vi "detector_acquire_generic_data.vi"(8 "error in (no error)":errorcluster, 11 "picoquant_generic in":refnum<class "picoquant_generic.lvclass">) -> (0 "error out":errorcluster, 2 "image_data":T1, 3 "picoquant_generic out":refnum<class "picoquant_generic.lvclass">)   [LabVIEW 2015, in "picoquant_generic.lvclass"]
uses:
  picoquant_generic.lvclass
  Experiment/experiment_panel/2d_scan/detector_data_tdef.ctl
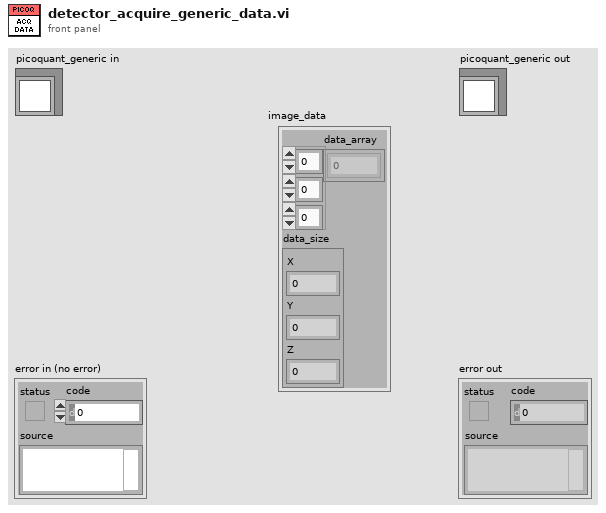
[diagram p1: front panel]
types:
  T1 = typedef "detector_data_tdef.ctl" = cluster{"data_array":dbl[][][], "data_size":cluster{"X":i32, "Y":i32, "Z":i32}}
  T2 = typedef "hydraharp_count_rates.ctl" = cluster{"channel_rates":i32[], "sync_rate":i32}
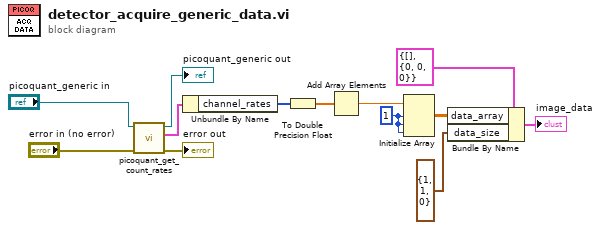
[diagram p0: block diagram]
diagram:
  w1 = 1 ("dimension size")
  n1 = call-dynamic "picoquant_get_count_rates.vi"("error in (no error)"="error in (no error)", "picoquant_generic in"="picoquant_generic in") -> ("error out"=→"error out":errorcluster, "count_rates"=w10:T2, "picoquant_generic out"=→"picoquant_generic out":refnum<class "picoquant_generic.lvclass">)  [unwired: 7 in]
  n2 = Unbundle By Name(w10) -> ("channel_rates"=w9:i32[])
  n3 = To Double Precision Float(number=w9) -> (double precision float=w8:dbl[])
  n4 = Add Array Elements(numeric array=w8) -> (sum=w2:dbl)
  n5 = Initialize Array(w2, w1, w1, w1) -> (w3:dbl[][][])
  n6 = Bundle By Name(cluster=T1 {"data_array"=[], "data_size"={"X"=0, "Y"=0, "Z"=0}} ("image_data"), "data_array"=w3, "data_size"=cluster{"X":i32, "Y":i32, "Z":i32} {"X"=1, "Y"=1, "Z"=0}) -> (→"image_data":T1)
